vi "AlGaInPAs_prep_run_cont_dil_v16.vi"(2 "Debug Mode":bool, 3 "Elapsed Time(s)":dbl, 4 "State":enum16{"Edit", "Start", "Run", "End", "Idle"}(ring), 5 "Argument List In":string[](array[string])) -> (0 "Status Out":string, 1 "Argument List Out":string[](array[string]))   [LabVIEW 2011]
panel:
  out "Ga calculated var":u16(ring)=1 items=["Ga flow", "MFC1", "MFC2", "MFC3"]
  out "GAMFC3 var":dbl=100.0 caption="R3 (0-1000 sscm)" format="%.1f"
  out "GAMFC2 var":dbl=10.0 caption="R2 (0-100 sscm)" format="%.2f"
  out "GAMFC1 var":dbl=1.0 caption="R1 (0-10 sscm)" format="%.2f"
  out "Ga Flow var":dbl=1.0 caption="Ga Flow (0-10 sscm)" format="%.4f"
  out "Prep-In var":bool
  out "Prep-Ga var":bool
  out "Prep-Al var":bool
  out "Prep-P var":bool
  out "Prep-As var":bool
  out "prep_done":bool
  out "run started":bool
  out "first":bool=TRUE
  out "total time":dbl
  out "is OK?":bool
  out "AsH3?":bool
  out "PH3?":bool
  out "In?":bool
  out "Ga?":bool
  out "Al?":bool
  in  "Prep As":bool caption="Pre-run"
  in  "Prep P":bool caption="Pre-run"
  in  "Prep In":bool caption="Pre-run"
  in  "prep_time":dbl caption="pre-run time (s)"
  in  "Prep Al":bool caption="Pre-run"
  in  "Run As":bool caption="Run"
  in  "AsH3 Flow":dbl caption="AsH3 Flow (0-10 sccm)" format="%.2f"
  in  "P Flow":dbl caption="P Flow (0-100 sccm)" format="%.2f"
  in  "Run P":bool caption="Run"
  in  "In Flow":dbl caption="In Flow (0-100 sscm)" format="%.2f"
  in  "Run In":bool caption="Run"
  in  "Run Al":bool caption="Run"
  in  "Al Flow":dbl caption="Al Flow (0-100 sscm)" format="%.2f"
  in  "Cancel":bool
  in  "OK":bool
  out "tTotal(s) 2":dbl
  in  "Ga Tab Control":enum32{"Page 1", "Page 2", "Page 3"}(tab)
  in  "Ga Dilution":bool caption="Dilute"
  in  "Run Ga":bool caption="Run"
  in  "Prep Ga":bool caption="Pre-run"
  out "Ga Flow val":dbl=1.0 caption="Ga Flow (0-10 sscm)" format="%.4f"
  in  "Ga Flow set":dbl=1.0 caption="Ga Flow (0-10 sscm)" format="%.4f"
  out "GAMFC1 val":dbl=1.0 caption="R1 (0-10 sscm)" format="%.2f"
  out "GAMFC3 val":dbl=100.0 caption="R3 (0-1000 sscm)" format="%.1f"
  out "GAMFC2 val":dbl=10.0 caption="R2 (0-100 sscm)" format="%.2f"
  in  "GAMFC1 set":dbl=1.0 caption="R1 (0-10 sscm)" format="%.2f"
  in  "GAMFC2 set":dbl=10.0 caption="R2 (0-100 sscm)" format="%.2f"
  in  "GAMFC3 set":dbl=100.0 caption="R3 (0-1000 sscm)" format="%.1f"
  in  "Ga calculated":u16(ring)=1 items=["Ga flow", "MFC1", "MFC2", "MFC3"]
  # "Add pre-run time to run time in editor."
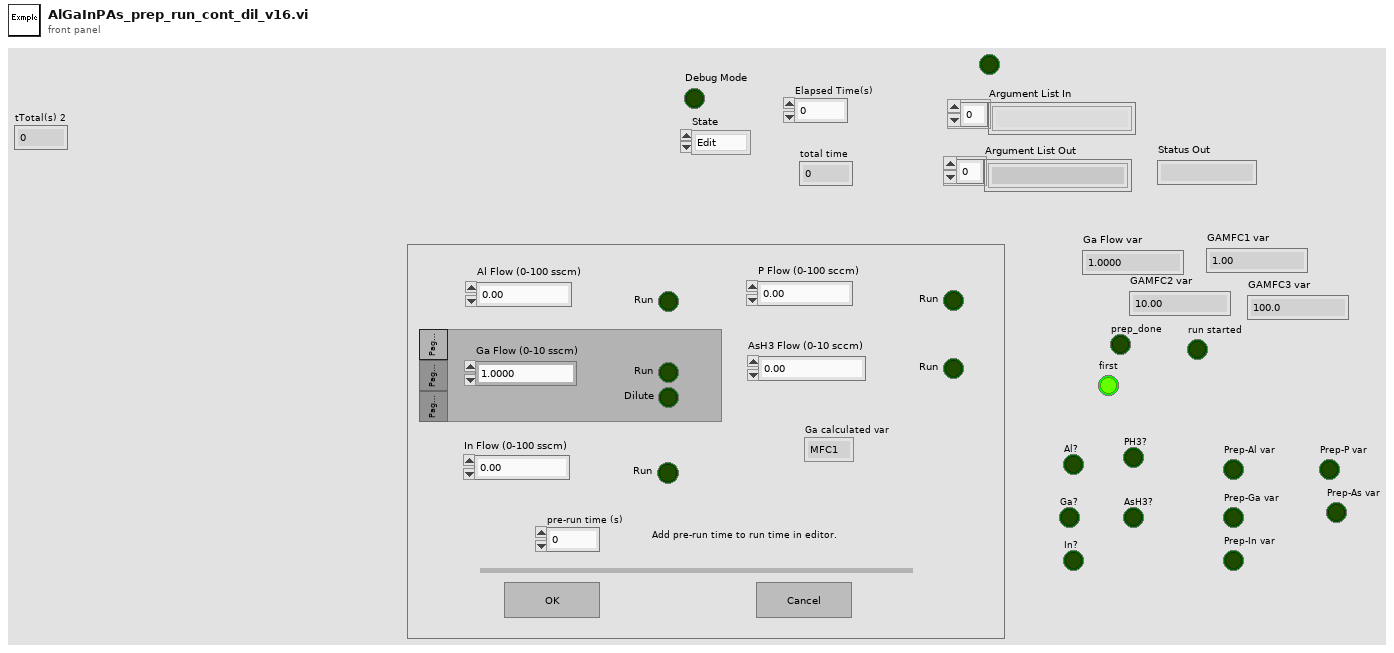
[diagram p1: front panel]
types:
  T1 = enum16{"Discrete", "Continuous", "Instantaneous", "Finite"}
  T2 = enum32{"Invalid", "Default", "Floating", "Floating/Auto-Hide", "Modal"}
  T3 = cluster{"Ga val":bool, "MFC1 val":bool, "MFC2 val":bool, "MFC3 val":bool, "Ga set":bool, "MFC1 set":bool, "MFC2 set":bool, "MFC3 set":bool}
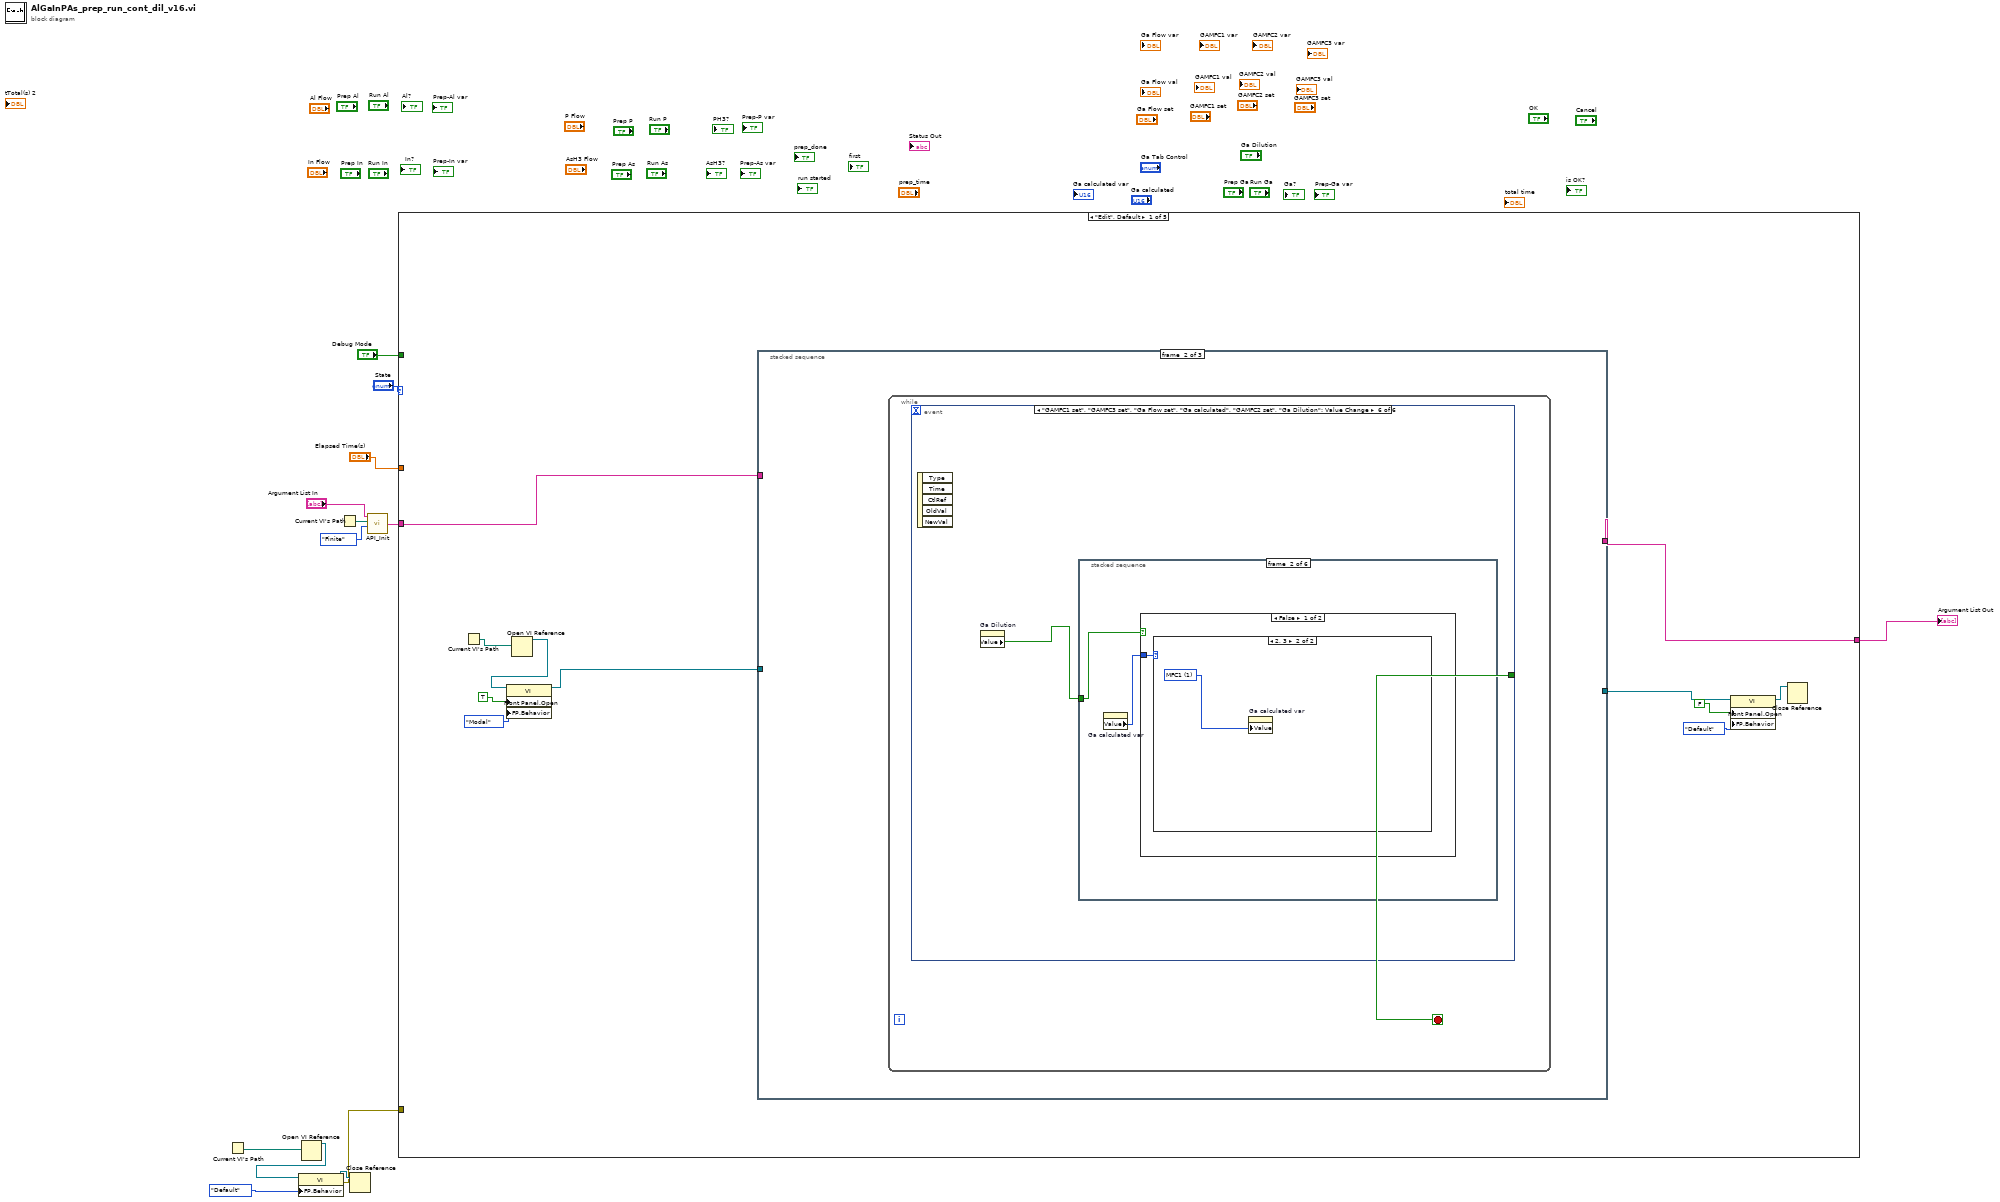
[diagram p0: block diagram]
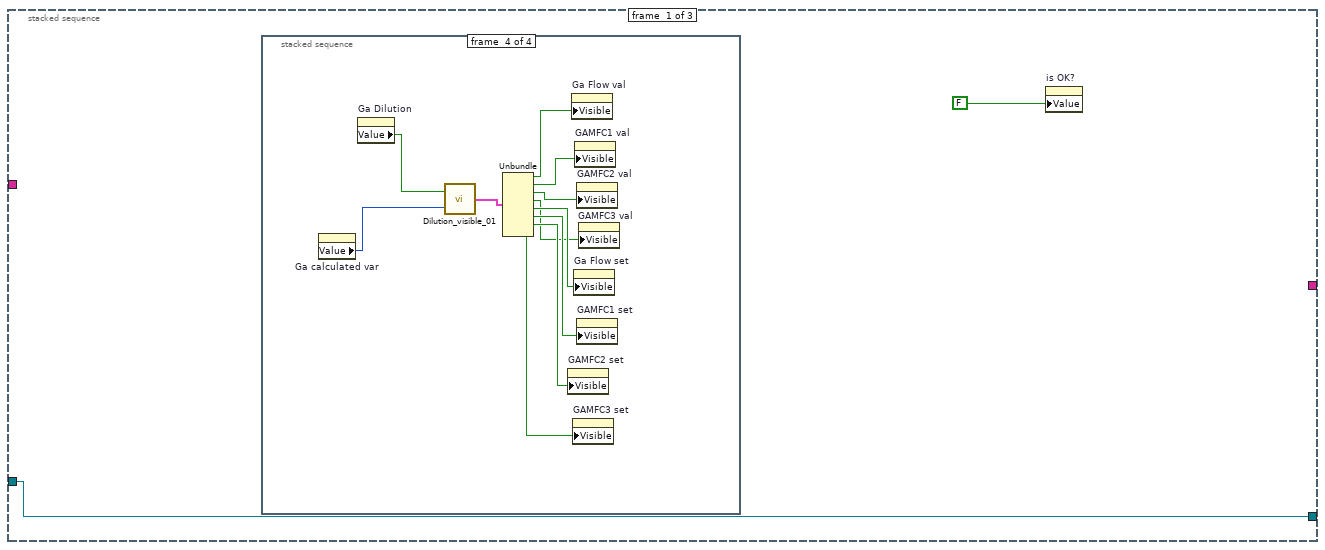
[diagram p2: hidden frame]
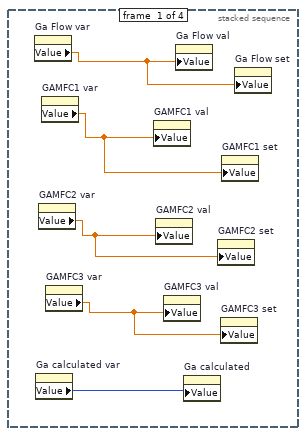
[diagram p3: hidden frame]
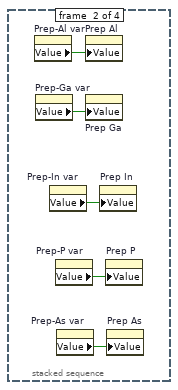
[diagram p4: hidden frame]
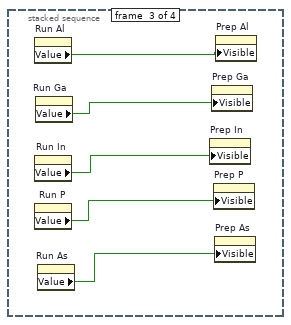
[diagram p5: hidden frame]
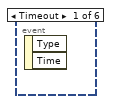
[diagram p6: hidden frame]
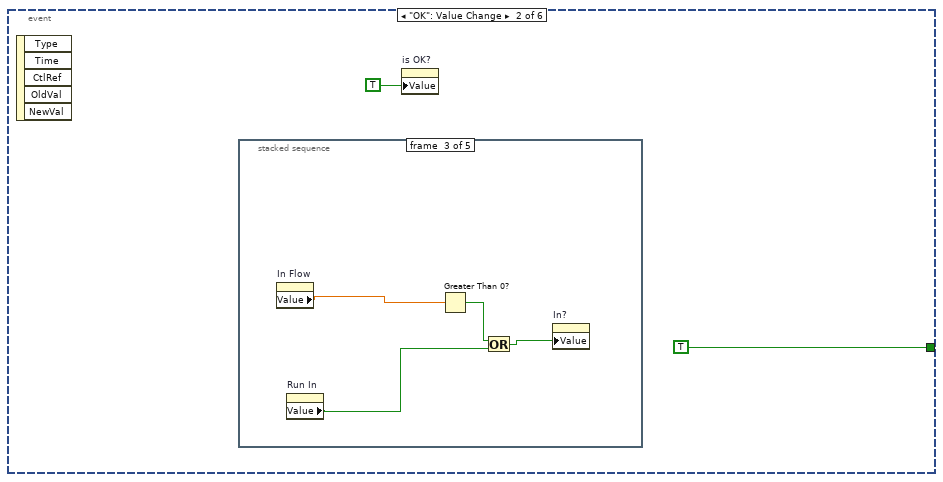
[diagram p7: hidden frame]
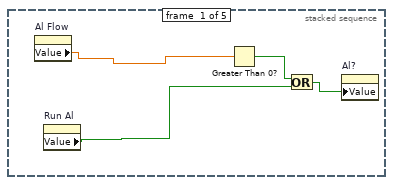
[diagram p8: hidden frame]
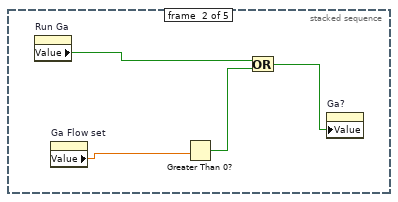
[diagram p9: hidden frame]
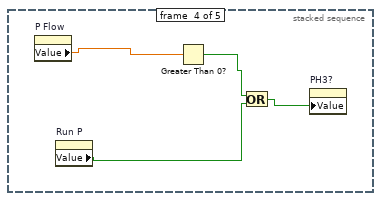
[diagram p10: hidden frame]
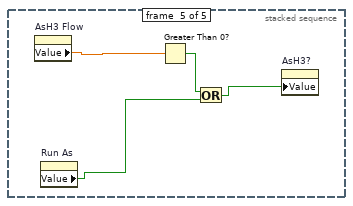
[diagram p11: hidden frame]
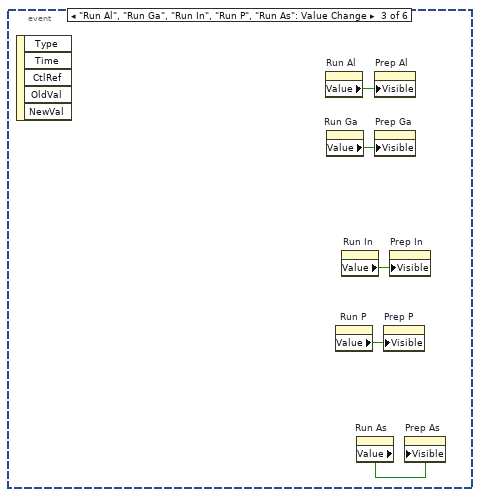
[diagram p12: hidden frame]
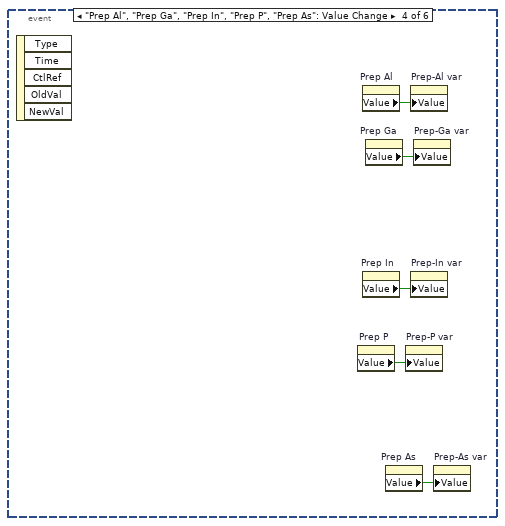
[diagram p13: hidden frame]
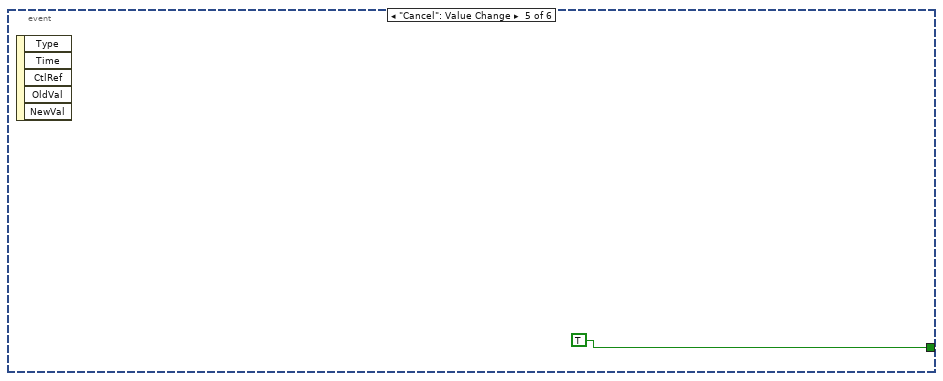
[diagram p14: hidden frame]
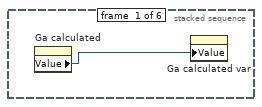
[diagram p15: hidden frame]
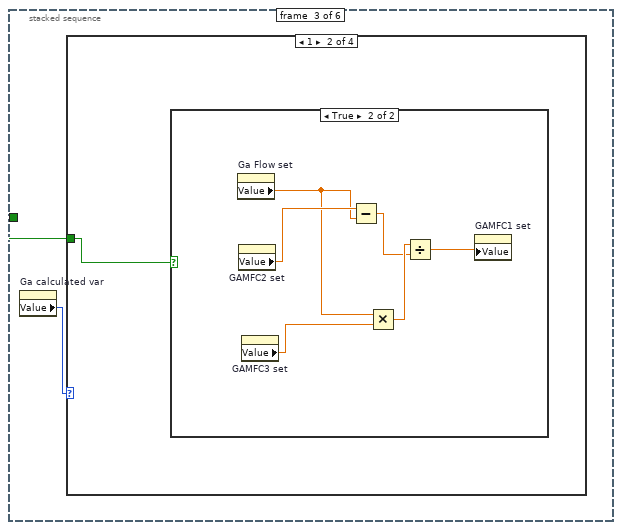
[diagram p18: hidden frame]
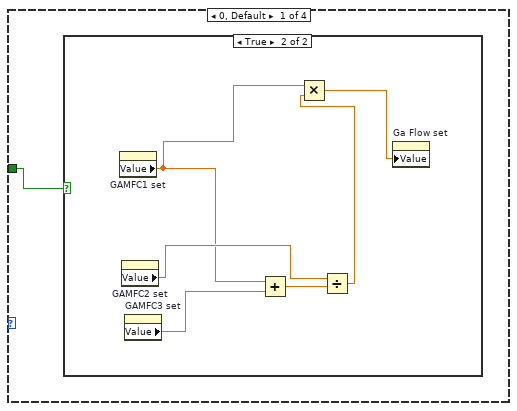
[diagram p19: hidden frame]
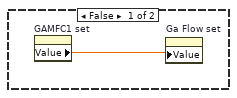
[diagram p20: hidden frame]
diagram:
  n1 = Current VI's Path() -> (path=w9:path)
  n2 = Open VI Reference(vi path=w9) -> (vi reference=w8:refnum<vi>)  [unwired: 1 in, 5 out]
  n3 = property class="VI"(reference=w8, "FP.Behavior"=T2."Default" ("Front Panel Window:Behavior")) -> (reference out=w6:refnum<vi>, error out=w5:errorcluster)  [unwired: 1 in]
  n4 = Current VI's Path() -> (path=w4:path)
  n5 = Close Reference(reference=w6) -> ()  [unwired: 1 in, 1 out]
  n6 = call "API_Init.vi"("API Mode"=T1."Finite", "VI Path"=w4, "Argument List In"="Argument List In") -> ("Argument List Out"=w1:string[])  [unwired: 1 in]
  n7 = case shown="\"Edit\", Default" "State" {
    tunnel: "Debug Mode" -> [_ w152 w206 _ _]
    tunnel: "Elapsed Time(s)" -> [_ _ w208 _ _]
    tunnel: w1 -> [w15 w154 w205 w323 w324]
    tunnel: [w14 w153 w207 w323 w324] -> w10
    tunnel: w5 -> [_ _ _ _ _]
    frame "Edit", Default {
      n8 = Current VI's Path() -> (path=w20:path)
      n9 = Open VI Reference(vi path=w20) -> (vi reference=w19:refnum<vi>)  [unwired: 1 in, 5 out]
      n10 = property class="VI"(reference=w19, "Front Panel.Open"=TRUE ("Front Panel Window:Open"), "FP.Behavior"=T2."Modal" ("Front Panel Window:Behavior")) -> (reference out=w18:refnum<vi>)  [unwired: 1 in, 1 out]
      n11 = stacked-sequence {
        tunnel: w15 -> [_ _ w147]
        tunnel: w18 -> [w26 _ _]
        tunnel: [w26 _ _] -> w22
        tunnel: [_ _ w145] -> w14
        frame #0 {
          n12 = stacked-sequence {
            frame #0 {
              n13 = property on="Ga Flow var" class="DigNum (strict)"() -> ("Value"=w31:dbl)  [unwired: 2 in, 2 out]
              n14 = property on="Ga calculated var" class="Ring (strict)"() -> ("Value"=w27:u16)  [unwired: 2 in, 2 out]
              n15 = property on="GAMFC2 var" class="DigNum (strict)"() -> ("Value"=w29:dbl)  [unwired: 2 in, 2 out]
              n16 = property on="GAMFC1 var" class="DigNum (strict)"() -> ("Value"=w28:dbl)  [unwired: 2 in, 2 out]
              n17 = property on="GAMFC3 var" class="DigNum (strict)"() -> ("Value"=w30:dbl)  [unwired: 2 in, 2 out]
              n18 = property on="GAMFC1 val" class="DigNum (strict)"("Value"=w28) -> ()  [unwired: 2 in, 2 out]
              n19 = property on="GAMFC2 val" class="DigNum (strict)"("Value"=w29) -> ()  [unwired: 2 in, 2 out]
              n20 = property on="GAMFC3 val" class="DigNum (strict)"("Value"=w30) -> ()  [unwired: 2 in, 2 out]
              n21 = property on="Ga Flow val" class="DigNum (strict)"("Value"=w31) -> ()  [unwired: 2 in, 2 out]
              n22 = property on="Ga calculated" class="Ring (strict)"("Value"=w27) -> ()  [unwired: 2 in, 2 out]
              n23 = property on="GAMFC2 set" class="DigNum (strict)"("Value"=w29) -> ()  [unwired: 2 in, 2 out]
              n24 = property on="GAMFC3 set" class="DigNum (strict)"("Value"=w30) -> ()  [unwired: 2 in, 2 out]
              n25 = property on="GAMFC1 set" class="DigNum (strict)"("Value"=w28) -> ()  [unwired: 2 in, 2 out]
              n26 = property on="Ga Flow set" class="DigNum (strict)"("Value"=w31) -> ()  [unwired: 2 in, 2 out]
            }
            frame #1 {
              n27 = property on="Prep-Al var" class="Bool (strict)"() -> ("Value"=w36:bool)  [unwired: 2 in, 2 out]
              n28 = property on="Prep-Ga var" class="Bool (strict)"() -> ("Value"=w35:bool)  [unwired: 2 in, 2 out]
              n29 = property on="Prep-In var" class="Bool (strict)"() -> ("Value"=w34:bool)  [unwired: 2 in, 2 out]
              n30 = property on="Prep-P var" class="Bool (strict)"() -> ("Value"=w33:bool)  [unwired: 2 in, 2 out]
              n31 = property on="Prep-As var" class="Bool (strict)"() -> ("Value"=w32:bool)  [unwired: 2 in, 2 out]
              n32 = property on="Prep Al" class="Bool (strict)"("Value"=w36) -> ()  [unwired: 2 in, 2 out]
              n33 = property on="Prep Ga" class="Bool (strict)"("Value"=w35) -> ()  [unwired: 2 in, 2 out]
              n34 = property on="Prep In" class="Bool (strict)"("Value"=w34) -> ()  [unwired: 2 in, 2 out]
              n35 = property on="Prep P" class="Bool (strict)"("Value"=w33) -> ()  [unwired: 2 in, 2 out]
              n36 = property on="Prep As" class="Bool (strict)"("Value"=w32) -> ()  [unwired: 2 in, 2 out]
            }
            frame #2 {
              n37 = property on="Run Al" class="Bool (strict)"() -> ("Value"=w41:bool)  [unwired: 2 in, 2 out]
              n38 = property on="Run In" class="Bool (strict)"() -> ("Value"=w39:bool)  [unwired: 2 in, 2 out]
              n39 = property on="Run P" class="Bool (strict)"() -> ("Value"=w38:bool)  [unwired: 2 in, 2 out]
              n40 = property on="Run Ga" class="Bool (strict)"() -> ("Value"=w40:bool)  [unwired: 2 in, 2 out]
              n41 = property on="Run As" class="Bool (strict)"() -> ("Value"=w37:bool)  [unwired: 2 in, 2 out]
              n42 = property on="Prep In" class="Bool (strict)"("Visible"=w39) -> ()  [unwired: 2 in, 2 out]
              n43 = property on="Prep Ga" class="Bool (strict)"("Visible"=w40) -> ()  [unwired: 2 in, 2 out]
              n44 = property on="Prep P" class="Bool (strict)"("Visible"=w38) -> ()  [unwired: 2 in, 2 out]
              n45 = property on="Prep As" class="Bool (strict)"("Visible"=w37) -> ()  [unwired: 2 in, 2 out]
              n46 = property on="Prep Al" class="Bool (strict)"("Visible"=w41) -> ()  [unwired: 2 in, 2 out]
            }
            frame #3 {
              n47 = property on="Ga calculated var" class="Ring (strict)"() -> ("Value"=w52:u16)  [unwired: 2 in, 2 out]
              n48 = property on="Ga Dilution" class="Bool (strict)"() -> ("Value"=w51:bool)  [unwired: 2 in, 2 out]
              n49 = call "Dilution_visible_01.vi"("calculated"=w52, "dilution"=w51) -> ("Visible"=w43:T3)
              n50 = Unbundle(w43) -> ("Ga val"=w44:bool, "MFC1 val"=w45:bool, "MFC2 val"=w42:bool, "MFC3 val"=w46:bool, "Ga set"=w47:bool, "MFC1 set"=w48:bool, "MFC2 set"=w49:bool, "MFC3 set"=w50:bool)
              n51 = property on="GAMFC2 set" class="DigNum (strict)"("Visible"=w49) -> ()  [unwired: 2 in, 2 out]
              n52 = property on="Ga Flow val" class="DigNum (strict)"("Visible"=w44) -> ()  [unwired: 2 in, 2 out]
              n53 = property on="GAMFC3 set" class="DigNum (strict)"("Visible"=w50) -> ()  [unwired: 2 in, 2 out]
              n54 = property on="Ga Flow set" class="DigNum (strict)"("Visible"=w47) -> ()  [unwired: 2 in, 2 out]
              n55 = property on="GAMFC1 val" class="DigNum (strict)"("Visible"=w45) -> ()  [unwired: 2 in, 2 out]
              n56 = property on="GAMFC2 val" class="DigNum (strict)"("Visible"=w42) -> ()  [unwired: 2 in, 2 out]
              n57 = property on="GAMFC1 set" class="DigNum (strict)"("Visible"=w48) -> ()  [unwired: 2 in, 2 out]
              n58 = property on="GAMFC3 val" class="DigNum (strict)"("Visible"=w46) -> ()  [unwired: 2 in, 2 out]
            }
          }
          n59 = property on="is OK?" class="Bool (strict)"("Value"=FALSE ("is OK?")) -> ()  [unwired: 2 in, 2 out]
        }
        frame #1 {
          n60 = while {
            stop <- w53 stop-if-true
            n61 = event shown="[5] \"GAMFC1 set\", \"GAMFC3 set\", \"Ga Flow set\", \"Ga calculated\", \"GAMFC2 set\", \"Ga Dilution\": Value Change" {
              selector: _ -> [_ _ _ _ _ _]
              dyn-events: _ -> [_ _ _ _ _ _]
              timeout: _ -> [_ _ _ _ _ _]
              tunnel: [_ TRUE _ _ TRUE _] -> w53
              event Timeout {
                n62 = event-data() -> ()  [unwired: 1 in, 2 out]
              }
              event "OK": Value Change {
                n63 = event-data() -> ()  [unwired: 1 in, 5 out]
                n64 = stacked-sequence {
                  frame #0 {
                    n65 = property on="Al Flow" class="DigNum (strict)"() -> ("Value"=w58:dbl)  [unwired: 2 in, 2 out]
                    n66 = property on="Run Al" class="Bool (strict)"() -> ("Value"=w57:bool)  [unwired: 2 in, 2 out]
                    n67 = Greater Than 0?(x=w58) -> (x > 0?=w59:bool)
                    n68 = Or(x=w59, y=w57) -> (x .or. y?=w56:bool)
                    n69 = property on="Al?" class="Bool (strict)"("Value"=w56) -> ()  [unwired: 2 in, 2 out]
                  }
                  frame #1 {
                    n70 = property on="Run Ga" class="Bool (strict)"() -> ("Value"=w61:bool)  [unwired: 2 in, 2 out]
                    n71 = property on="Ga Flow set" class="DigNum (strict)"() -> ("Value"=w62:dbl)  [unwired: 2 in, 2 out]
                    n72 = Greater Than 0?(x=w62) -> (x > 0?=w63:bool)
                    n73 = Or(x=w61, y=w63) -> (x .or. y?=w60:bool)
                    n74 = property on="Ga?" class="Bool (strict)"("Value"=w60) -> ()  [unwired: 2 in, 2 out]
                  }
                  frame #2 {
                    n75 = property on="In Flow" class="DigNum (strict)"() -> ("Value"=w65:dbl)  [unwired: 2 in, 2 out]
                    n76 = property on="Run In" class="Bool (strict)"() -> ("Value"=w66:bool)  [unwired: 2 in, 2 out]
                    n77 = Greater Than 0?(x=w65) -> (x > 0?=w67:bool)
                    n78 = Or(x=w67, y=w66) -> (x .or. y?=w64:bool)
                    n79 = property on="In?" class="Bool (strict)"("Value"=w64) -> ()  [unwired: 2 in, 2 out]
                  }
                  frame #3 {
                    n80 = property on="P Flow" class="DigNum (strict)"() -> ("Value"=w70:dbl)  [unwired: 2 in, 2 out]
                    n81 = property on="Run P" class="Bool (strict)"() -> ("Value"=w69:bool)  [unwired: 2 in, 2 out]
                    n82 = Greater Than 0?(x=w70) -> (x > 0?=w71:bool)
                    n83 = Or(x=w71, y=w69) -> (x .or. y?=w68:bool)
                    n84 = property on="PH3?" class="Bool (strict)"("Value"=w68) -> ()  [unwired: 2 in, 2 out]
                  }
                  frame #4 {
                    n85 = property on="AsH3 Flow" class="DigNum (strict)"() -> ("Value"=w74:dbl)  [unwired: 2 in, 2 out]
                    n86 = property on="Run As" class="Bool (strict)"() -> ("Value"=w73:bool)  [unwired: 2 in, 2 out]
                    n87 = Greater Than 0?(x=w74) -> (x > 0?=w75:bool)
                    n88 = Or(x=w75, y=w73) -> (x .or. y?=w72:bool)
                    n89 = property on="AsH3?" class="Bool (strict)"("Value"=w72) -> ()  [unwired: 2 in, 2 out]
                  }
                }
                n90 = property on="is OK?" class="Bool (strict)"("Value"=TRUE ("is OK?")) -> ()  [unwired: 2 in, 2 out]
              }
              event "Run Al", "Run Ga", "Run In", "Run P", "Run As": Value Change {
                n91 = event-data() -> ()  [unwired: 1 in, 5 out]
                n92 = property on="Run Al" class="Bool (strict)"() -> ("Value"=w80:bool)  [unwired: 2 in, 2 out]
                n93 = property on="Run Ga" class="Bool (strict)"() -> ("Value"=w79:bool)  [unwired: 2 in, 2 out]
                n94 = property on="Run P" class="Bool (strict)"() -> ("Value"=w76:bool)  [unwired: 2 in, 2 out]
                n95 = property on="Run In" class="Bool (strict)"() -> ("Value"=w78:bool)  [unwired: 2 in, 2 out]
                n96 = property on="Run As" class="Bool (strict)"() -> ("Value"=w77:bool)  [unwired: 2 in, 2 out]
                n97 = property on="Prep Al" class="Bool (strict)"("Visible"=w80) -> ()  [unwired: 2 in, 2 out]
                n98 = property on="Prep Ga" class="Bool (strict)"("Visible"=w79) -> ()  [unwired: 2 in, 2 out]
                n99 = property on="Prep P" class="Bool (strict)"("Visible"=w76) -> ()  [unwired: 2 in, 2 out]
                n100 = property on="Prep In" class="Bool (strict)"("Visible"=w78) -> ()  [unwired: 2 in, 2 out]
                n101 = property on="Prep As" class="Bool (strict)"("Visible"=w77) -> ()  [unwired: 2 in, 2 out]
              }
              event "Prep Al", "Prep Ga", "Prep In", "Prep P", "Prep As": Value Change {
                n102 = event-data() -> ()  [unwired: 1 in, 5 out]
                n103 = property on="Prep P" class="Bool (strict)"() -> ("Value"=w82:bool)  [unwired: 2 in, 2 out]
                n104 = property on="Prep Al" class="Bool (strict)"() -> ("Value"=w85:bool)  [unwired: 2 in, 2 out]
                n105 = property on="Prep In" class="Bool (strict)"() -> ("Value"=w83:bool)  [unwired: 2 in, 2 out]
                n106 = property on="Prep Ga" class="Bool (strict)"() -> ("Value"=w84:bool)  [unwired: 2 in, 2 out]
                n107 = property on="Prep As" class="Bool (strict)"() -> ("Value"=w81:bool)  [unwired: 2 in, 2 out]
                n108 = property on="Prep-P var" class="Bool (strict)"("Value"=w82) -> ()  [unwired: 2 in, 2 out]
                n109 = property on="Prep-Al var" class="Bool (strict)"("Value"=w85) -> ()  [unwired: 2 in, 2 out]
                n110 = property on="Prep-In var" class="Bool (strict)"("Value"=w83) -> ()  [unwired: 2 in, 2 out]
                n111 = property on="Prep-Ga var" class="Bool (strict)"("Value"=w84) -> ()  [unwired: 2 in, 2 out]
                n112 = property on="Prep-As var" class="Bool (strict)"("Value"=w81) -> ()  [unwired: 2 in, 2 out]
              }
              event "Cancel": Value Change {
                n113 = event-data() -> ()  [unwired: 1 in, 5 out]
              }
              event "GAMFC1 set", "GAMFC3 set", "Ga Flow set", "Ga calculated", "GAMFC2 set", "Ga Dilution": Value Change {
                n114 = event-data() -> ()  [unwired: 1 in, 5 out]
                n115 = property on="Ga Dilution" class="Bool (strict)"() -> ("Value"=w87:bool)  [unwired: 2 in, 2 out]
                n116 = stacked-sequence {
                  tunnel: w87 -> [_ w90 w94 w135 _ w141]
                  frame #0 {
                    n117 = property on="Ga calculated" class="Ring (strict)"() -> ("Value"=w88:u16)  [unwired: 2 in, 2 out]
                    n118 = property on="Ga calculated var" class="Ring (strict)"("Value"=w88) -> ()  [unwired: 2 in, 2 out]
                  }
                  frame #1 {
                    n119 = property on="Ga calculated var" class="Ring (strict)"() -> ("Value"=w89:u16)  [unwired: 2 in, 2 out]
                    n120 = case shown="False" w90 {
                      tunnel: w89 -> [w91 _]
                      frame False {
                        n121 = case shown="2, 3" w91 {
                          frame 0, 1, Default {
                          }
                          frame 2, 3 {
                            w92 = u16 1 items=["Ga flow", "MFC1", "MFC2", "MFC3"] ("Ga calculated")
                            n122 = property on="Ga calculated var" class="Ring (strict)"("Value"=w92) -> ()  [unwired: 2 in, 2 out]
                          }
                        }
                      }
                      frame True {
                      }
                    }
                  }
                  frame #2 {
                    n123 = property on="Ga calculated var" class="Ring (strict)"() -> ("Value"=w93:u16)  [unwired: 2 in, 2 out]
                    n124 = case shown="1" w93 {
                      tunnel: w94 -> [w95 w103 w111 w118]
                      frame 0, Default {
                        n125 = case shown="True" w95 {
                          frame False {
                            n126 = property on="GAMFC1 set" class="DigNum (strict)"() -> ("Value"=w96:dbl)  [unwired: 2 in, 2 out]
                            n127 = property on="Ga Flow set" class="DigNum (strict)"("Value"=w96) -> ()  [unwired: 2 in, 2 out]
                          }
                          frame True {
                            n128 = property on="GAMFC1 set" class="DigNum (strict)"() -> ("Value"=w98:dbl)  [unwired: 2 in, 2 out]
                            n129 = property on="GAMFC2 set" class="DigNum (strict)"() -> ("Value"=w100:dbl)  [unwired: 2 in, 2 out]
                            n130 = property on="GAMFC3 set" class="DigNum (strict)"() -> ("Value"=w102:dbl)  [unwired: 2 in, 2 out]
                            n131 = Add(x=w98, y=w102) -> (x+y=w101:dbl)
                            n132 = Divide(x=w100, y=w101) -> (x/y=w99:dbl)
                            n133 = Multiply(x=w98, y=w99) -> (x*y=w97:dbl)
                            n134 = property on="Ga Flow set" class="DigNum (strict)"("Value"=w97) -> ()  [unwired: 2 in, 2 out]
                          }
                        }
                      }
                      frame 1 {
                        n135 = case shown="True" w103 {
                          frame False {
                            n136 = property on="Ga Flow set" class="DigNum (strict)"() -> ("Value"=w104:dbl)  [unwired: 2 in, 2 out]
                            n137 = property on="GAMFC1 set" class="DigNum (strict)"("Value"=w104) -> ()  [unwired: 2 in, 2 out]
                          }
                          frame True {
                            n138 = property on="Ga Flow set" class="DigNum (strict)"() -> ("Value"=w109:dbl)  [unwired: 2 in, 2 out]
                            n139 = property on="GAMFC2 set" class="DigNum (strict)"() -> ("Value"=w110:dbl)  [unwired: 2 in, 2 out]
                            n140 = property on="GAMFC3 set" class="DigNum (strict)"() -> ("Value"=w108:dbl)  [unwired: 2 in, 2 out]
                            n141 = Subtract(x=w110, y=w109) -> (x-y=w106:dbl)
                            n142 = Multiply(x=w109, y=w108) -> (x*y=w107:dbl)
                            n143 = Divide(x=w107, y=w106) -> (x/y=w105:dbl)
                            n144 = property on="GAMFC1 set" class="DigNum (strict)"("Value"=w105) -> ()  [unwired: 2 in, 2 out]
                          }
                        }
                      }
                      frame 2 {
                        n145 = case shown="True" w111 {
                          frame False {
                          }
                          frame True {
                            n146 = property on="GAMFC1 set" class="DigNum (strict)"() -> ("Value"=w113:dbl)  [unwired: 2 in, 2 out]
                            n147 = property on="GAMFC3 set" class="DigNum (strict)"() -> ("Value"=w115:dbl)  [unwired: 2 in, 2 out]
                            n148 = property on="Ga Flow set" class="DigNum (strict)"() -> ("Value"=w116:dbl)  [unwired: 2 in, 2 out]
                            n149 = Add(x=w113, y=w115) -> (x+y=w117:dbl)
                            n150 = Multiply(x=w116, y=w117) -> (x*y=w114:dbl)
                            n151 = Divide(x=w114, y=w113) -> (x/y=w112:dbl)
                            n152 = property on="GAMFC2 set" class="DigNum (strict)"("Value"=w112) -> ()  [unwired: 2 in, 2 out]
                          }
                        }
                      }
                      frame 3 {
                        n153 = case shown="True" w118 {
                          frame False {
                          }
                          frame True {
                            n154 = property on="GAMFC2 set" class="DigNum (strict)"() -> ("Value"=w124:dbl)  [unwired: 2 in, 2 out]
                            n155 = property on="Ga Flow set" class="DigNum (strict)"() -> ("Value"=w122:dbl)  [unwired: 2 in, 2 out]
                            n156 = property on="GAMFC1 set" class="DigNum (strict)"() -> ("Value"=w123:dbl)  [unwired: 2 in, 2 out]
                            n157 = Subtract(x=w124, y=w122) -> (x-y=w120:dbl)
                            n158 = Divide(x=w123, y=w122) -> (x/y=w121:dbl)
                            n159 = Multiply(x=w121, y=w120) -> (x*y=w119:dbl)
                            n160 = property on="GAMFC3 set" class="DigNum (strict)"("Value"=w119) -> ()  [unwired: 2 in, 2 out]
                          }
                        }
                      }
                    }
                  }
                  frame #3 {
                    n161 = property on="Ga calculated var" class="Ring (strict)"() -> ("Value"=w125:u16)  [unwired: 2 in, 2 out]
                    n162 = call "Dilution_visible_01.vi"("calculated"=w125, "dilution"=w135) -> ("Visible"=w131:T3)
                    n163 = Unbundle(w131) -> ("Ga val"=w134:bool, "MFC1 val"=w133:bool, "MFC2 val"=w132:bool, "MFC3 val"=w130:bool, "Ga set"=w129:bool, "MFC1 set"=w128:bool, "MFC2 set"=w127:bool, "MFC3 set"=w126:bool)
                    n164 = property on="Ga Flow set" class="DigNum (strict)"("Visible"=w129) -> ()  [unwired: 2 in, 2 out]
                    n165 = property on="GAMFC1 set" class="DigNum (strict)"("Visible"=w128) -> ()  [unwired: 2 in, 2 out]
                    n166 = property on="GAMFC3 set" class="DigNum (strict)"("Visible"=w126) -> ()  [unwired: 2 in, 2 out]
                    n167 = property on="GAMFC2 set" class="DigNum (strict)"("Visible"=w127) -> ()  [unwired: 2 in, 2 out]
                    n168 = property on="Ga Flow val" class="DigNum (strict)"("Visible"=w134) -> ()  [unwired: 2 in, 2 out]
                    n169 = property on="GAMFC1 val" class="DigNum (strict)"("Visible"=w133) -> ()  [unwired: 2 in, 2 out]
                    n170 = property on="GAMFC2 val" class="DigNum (strict)"("Visible"=w132) -> ()  [unwired: 2 in, 2 out]
                    n171 = property on="GAMFC3 val" class="DigNum (strict)"("Visible"=w130) -> ()  [unwired: 2 in, 2 out]
                  }
                  frame #4 {
                    n172 = property on="GAMFC1 set" class="DigNum (strict)"() -> ("Value"=w139:dbl)  [unwired: 2 in, 2 out]
                    n173 = property on="Ga Flow set" class="DigNum (strict)"() -> ("Value"=w140:dbl)  [unwired: 2 in, 2 out]
                    n174 = property on="GAMFC2 set" class="DigNum (strict)"() -> ("Value"=w138:dbl)  [unwired: 2 in, 2 out]
                    n175 = property on="GAMFC3 set" class="DigNum (strict)"() -> ("Value"=w137:dbl)  [unwired: 2 in, 2 out]
                    n176 = property on="Ga calculated var" class="Ring (strict)"() -> ("Value"=w136:u16)  [unwired: 2 in, 2 out]
                    n177 = property on="GAMFC3 val" class="DigNum (strict)"("Value"=w137) -> ()  [unwired: 2 in, 2 out]
                    n178 = property on="GAMFC1 val" class="DigNum (strict)"("Value"=w139) -> ()  [unwired: 2 in, 2 out]
                    n179 = property on="GAMFC2 val" class="DigNum (strict)"("Value"=w138) -> ()  [unwired: 2 in, 2 out]
                    n180 = property on="Ga Flow val" class="DigNum (strict)"("Value"=w140) -> ()  [unwired: 2 in, 2 out]
                    n181 = property on="Ga calculated" class="Ring (strict)"("Value"=w136) -> ()  [unwired: 2 in, 2 out]
                    n182 = property on="GAMFC3 var" class="DigNum (strict)"("Value"=w137) -> ()  [unwired: 2 in, 2 out]
                    n183 = property on="GAMFC1 var" class="DigNum (strict)"("Value"=w139) -> ()  [unwired: 2 in, 2 out]
                    n184 = property on="GAMFC2 var" class="DigNum (strict)"("Value"=w138) -> ()  [unwired: 2 in, 2 out]
                    n185 = property on="Ga Flow var" class="DigNum (strict)"("Value"=w140) -> ()  [unwired: 2 in, 2 out]
                  }
                  frame #5 {
                    n186 = case shown="False" w141 {
                      frame False {
                        n187 = property on="Ga calculated" class="Ring (strict)"("Disabled Items []"=i32[] [2, 3]) -> ()  [unwired: 2 in, 2 out]
                      }
                      frame True {
                        n188 = property on="Ga calculated" class="Ring (strict)"("Disabled Items []"=i32[] []) -> ()  [unwired: 2 in, 2 out]
                      }
                    }
                  }
                }
              }
            }
          }
        }
        frame #2 {
          n189 = property on="is OK?" class="Bool (strict)"() -> ("Value"=w144:bool)  [unwired: 2 in, 2 out]
          n190 = case shown="True" w144 {
            tunnel: w147 -> [w150 w151]
            tunnel: [w150 w151] -> w146
            frame False {
            }
            frame True {
            }
          }
          n191 = Not(x=w144) -> (.not. x?=w149:bool)
          n192 = Current VI's Path() -> (path=w148:path)
          n193 = call "API_Edit.vi"("Cancel"=w149, "OK"=w144, "VI Path"=w148, "Argument List In"=w146) -> ("Argument List Out"=w145:string[])
        }
      }
      n194 = property class="VI"(reference=w22, "Front Panel.Open"=FALSE ("Front Panel Window:Open"), "FP.Behavior"=T2."Default" ("Front Panel Window:Behavior")) -> (reference out=w23:refnum<vi>)  [unwired: 1 in, 1 out]
      n195 = Close Reference(reference=w23) -> ()  [unwired: 1 in, 1 out]
    }
    frame "Start" {
      n196 = call "Set_Argument.vi"("Enable"=FALSE, "Argument"="run_started", "Argument List In"=w154) -> ("Argument List Out"=w153:string[])
      n197 = stacked-sequence {
        tunnel: w152 -> [w157 w166 w178 w187 w196]
        frame #0 {
          n198 = case shown="False" w157 {
            frame False {
              n199 = property on="Al?" class="Bool (strict)"() -> ("Value"=w158:bool)  [unwired: 2 in, 2 out]
              n200 = case shown="True" w158 {
                frame False {
                  w159 = FALSE ("Al Active")
                  n201 = call "set_Al.vi"("Aluminum Flow"=0.0, "Al Remote"=w159, "Al Run"=w159, "Al Bubbler"=w159, "Al Active"=w159) -> ()  [unwired: 5 out]
                }
                frame True {
                  w165 = TRUE ("Al Active")
                  n202 = property on="Prep Al" class="Bool (strict)"() -> ("Value"=w163:bool)  [unwired: 2 in, 2 out]
                  n203 = property on="Run Al" class="Bool (strict)"() -> ("Value"=w162:bool)  [unwired: 2 in, 2 out]
                  n204 = property on="Al Flow" class="DigNum (strict)"() -> ("Value"=w164:dbl)  [unwired: 2 in, 2 out]
                  n205 = And(x=w163, y=w162) -> (x .and. y?=w161:bool)
                  n206 = call "set_Al.vi"("Aluminum Flow"=w164, "Al Run"=w161, "Al Bubbler"=w165, "Al Active"=w165) -> ()  [unwired: 1 in, 5 out]
                }
              }
            }
            frame True {
            }
          }
        }
        frame #1 {
          n207 = case shown="False" w166 {
            frame False {
              n208 = property on="Ga?" class="Bool (strict)"() -> ("Value"=w167:bool)  [unwired: 2 in, 2 out]
              n209 = case shown="True" w167 {
                frame False {
                  w169 = FALSE ("Ga Active")
                  w168 = 0.0 ("Ga Flow 1")
                  n210 = call "set_Ga.vi"("Ga Active"=w169, "Ga Flow 3"=w168, "Ga Flow 2"=w168, "Ga Flow 1"=w168, "Ga Bubbler"=w169, "Ga H2 Dilute"=w169, "Ga Run"=w169, "Ga Remote"=w169) -> ()  [unwired: 8 out]
                }
                frame True {
                  w173 = TRUE ("Ga Active")
                  n211 = property on="GAMFC3 var" class="DigNum (strict)"() -> ("Value"=w170:dbl)  [unwired: 2 in, 2 out]
                  n212 = property on="GAMFC2 var" class="DigNum (strict)"() -> ("Value"=w171:dbl)  [unwired: 2 in, 2 out]
                  n213 = property on="GAMFC1 var" class="DigNum (strict)"() -> ("Value"=w172:dbl)  [unwired: 2 in, 2 out]
                  n214 = property on="Prep-Ga var" class="Bool (strict)"() -> ("Value"=w174:bool)  [unwired: 2 in, 2 out]
                  n215 = property on="Run Ga" class="Bool (strict)"() -> ("Value"=w175:bool)  [unwired: 2 in, 2 out]
                  n216 = And(x=w174, y=w175) -> (x .and. y?=w177:bool)
                  n217 = property on="Ga Dilution" class="Bool (strict)"() -> ("Value"=w176:bool)  [unwired: 2 in, 2 out]
                  n218 = call "set_Ga.vi"("Ga Active"=w173, "Ga Flow 3"=w170, "Ga Flow 2"=w171, "Ga Flow 1"=w172, "Ga Bubbler"=w173, "Ga H2 Dilute"=w176, "Ga Run"=w177, "Ga Remote"=w173) -> ()  [unwired: 8 in]
                }
              }
            }
            frame True {
            }
          }
        }
        frame #2 {
          n219 = case shown="False" w178 {
            frame False {
              n220 = property on="In?" class="Bool (strict)"() -> ("Value"=w179:bool)  [unwired: 2 in, 2 out]
              n221 = case shown="True" w179 {
                frame False {
                  w181 = FALSE ("In Remote")
                  n222 = call "set_In.vi"("Indium Flow"=0.0, "In Remote"=w181, "In Run"=w181, "In Bubbler"=w181, "In Active"=w181) -> ()  [unwired: 5 out]
                }
                frame True {
                  w186 = TRUE ("In Run")
                  n223 = property on="Run In" class="Bool (strict)"() -> ("Value"=w183:bool)  [unwired: 2 in, 2 out]
                  n224 = property on="Prep In" class="Bool (strict)"() -> ("Value"=w184:bool)  [unwired: 2 in, 2 out]
                  n225 = And(x=w184, y=w183) -> (x .and. y?=w182:bool)
                  n226 = property on="In Flow" class="DigNum (strict)"() -> ("Value"=w185:dbl)  [unwired: 2 in, 2 out]
                  n227 = call "set_In.vi"("Indium Flow"=w185, "In Run"=w182, "In Bubbler"=w186, "In Active"=w186) -> ()  [unwired: 1 in, 5 out]
                }
              }
            }
            frame True {
            }
          }
        }
        frame #3 {
          n228 = case shown="False" w187 {
            frame False {
              n229 = property on="PH3?" class="Bool (strict)"() -> ("Value"=w188:bool)  [unwired: 2 in, 2 out]
              n230 = case shown="True" w188 {
                frame False {
                  w189 = FALSE ("P_Gas Active")
                  n231 = call "set_P_gas.vi"("P_Gas Active"=w189, "P_Gas Flow"=0.0, "P_Gas In"=w189, "P_Gas H2 In"=w189, "P_Gas Run"=w189, "P_Gas Remote"=w189) -> ()  [unwired: 10 out]
                }
                frame True {
                  w195 = TRUE ("P_Gas Active")
                  n232 = property on="P Flow" class="DigNum (strict)"() -> ("Value"=w194:dbl)  [unwired: 2 in, 2 out]
                  n233 = property on="Prep P" class="Bool (strict)"() -> ("Value"=w193:bool)  [unwired: 2 in, 2 out]
                  n234 = property on="Run P" class="Bool (strict)"() -> ("Value"=w192:bool)  [unwired: 2 in, 2 out]
                  n235 = And(x=w193, y=w192) -> (x .and. y?=w191:bool)
                  n236 = call "set_P_gas.vi"("P_Gas Active"=w195, "P_Gas Flow"=w194, "P_Gas In"=w195, "P_Gas Run"=w191) -> ()  [unwired: 2 in, 10 out]
                }
              }
            }
            frame True {
            }
          }
        }
        frame #4 {
          n237 = case shown="False" w196 {
            frame False {
              n238 = property on="AsH3?" class="Bool (strict)"() -> ("Value"=w197:bool)  [unwired: 2 in, 2 out]
              n239 = case shown="True" w197 {
                frame False {
                  w198 = FALSE ("As_Gas Active")
                  n240 = call "set_As_gas.vi"("As_Gas Active"=w198, "As_Gas Flow"=0.0, "As_Gas In"=w198, "As_Gas H2"=w198, "As_Gas Run"=w198, "As_Gas Remote"=w198) -> ()  [unwired: 10 in]
                }
                frame True {
                  w204 = TRUE ("As_Gas Active")
                  n241 = property on="Prep As" class="Bool (strict)"() -> ("Value"=w201:bool)  [unwired: 2 in, 2 out]
                  n242 = property on="Run As" class="Bool (strict)"() -> ("Value"=w202:bool)  [unwired: 2 in, 2 out]
                  n243 = property on="AsH3 Flow" class="DigNum (strict)"() -> ("Value"=w203:dbl)  [unwired: 2 in, 2 out]
                  n244 = And(x=w201, y=w202) -> (x .and. y?=w200:bool)
                  n245 = call "set_As_gas.vi"("As_Gas Active"=w204, "As_Gas Flow"=w203, "As_Gas In"=w204, "As_Gas Run"=w200) -> ()  [unwired: 12 in]
                }
              }
            }
            frame True {
            }
          }
        }
      }
    }
    frame "Run" {
      n246 = stacked-sequence {
        tunnel: w208 -> [_ w213 _ _]
        tunnel: w205 -> [w210 _ _ w267]
        tunnel: [_ _ _ w266] -> w207
        tunnel: w206 -> [_ _ _ w268]
        frame #0 {
          n247 = call "Get_Argument.vi"("Argument"="run_started", "Argument List"=w210) -> ("Enabled"=w209:bool)
          n248 = local write "run started"(w209) -> ()
        }
        frame #1 {
          n249 = property on="prep_time" class="DigNum (strict)"() -> ("Value"=w214:dbl)  [unwired: 2 in, 2 out]
          n250 = Greater Or Equal?(x=w213, y=w214) -> (x >= y?=w212:bool)
          n251 = local write "prep_done"(w212) -> ()
        }
        frame #2 {
          n252 = local read "run started"() -> (w216:bool)
          n253 = Not(x=w216) -> (.not. x?=w215:bool)
          n254 = stacked-sequence {
            tunnel: w215 -> [w218 w222 w231 w240 w249 w258]
            frame #0 {
              n255 = case shown="True" w218 {
                tunnel: ["run: " "pre-run: "] -> w217
                frame False {
                }
                frame True {
                }
              }
              n256 = property on="Status Out" class="Str"("Value"=w217) -> ()  [unwired: 2 in, 2 out]
            }
            frame #1 {
              n257 = property on="Status Out" class="Str"() -> ("Value"=w228:string)  [unwired: 2 in, 2 out]
              n258 = property on="Al?" class="Bool (strict)"() -> ("Value"=w229:bool)  [unwired: 2 in, 2 out]
              n259 = property on="Run Al" class="Bool (strict)"() -> ("Value"=w221:bool)  [unwired: 2 in, 2 out]
              n260 = property on="Prep Al" class="Bool (strict)"() -> ("Value"=w223:bool)  [unwired: 2 in, 2 out]
              n261 = call "flow_strings.vi"("string in"=w228, "is first in?"=TRUE, "use source?"=w229, "name"="Al", "run source?"=w221, "prep source?"=w223, "is prep?"=w222) -> ("string out"=w227:string, "is first out?"=w226:bool)
              n262 = property on="Status Out" class="Str"("Value"=w227) -> ()  [unwired: 2 in, 2 out]
              n263 = property on="first" class="Bool (strict)"("Value"=w226) -> ()  [unwired: 2 in, 2 out]
            }
            frame #2 {
              n264 = property on="first" class="Bool (strict)"() -> ("Value"=w234:bool)  [unwired: 2 in, 2 out]
              n265 = property on="Status Out" class="Str"() -> ("Value"=w237:string)  [unwired: 2 in, 2 out]
              n266 = property on="Ga?" class="Bool (strict)"() -> ("Value"=w235:bool)  [unwired: 2 in, 2 out]
              n267 = property on="Run Ga" class="Bool (strict)"() -> ("Value"=w230:bool)  [unwired: 2 in, 2 out]
              n268 = property on="Prep Ga" class="Bool (strict)"() -> ("Value"=w232:bool)  [unwired: 2 in, 2 out]
              n269 = call "flow_strings.vi"("string in"=w237, "is first in?"=w234, "use source?"=w235, "name"="Ga", "run source?"=w230, "prep source?"=w232, "is prep?"=w231) -> ("string out"=w238:string, "is first out?"=w233:bool)
              n270 = property on="Status Out" class="Str"("Value"=w238) -> ()  [unwired: 2 in, 2 out]
              n271 = property on="first" class="Bool (strict)"("Value"=w233) -> ()  [unwired: 2 in, 2 out]
            }
            frame #3 {
              n272 = property on="first" class="Bool (strict)"() -> ("Value"=w244:bool)  [unwired: 2 in, 2 out]
              n273 = property on="Status Out" class="Str"() -> ("Value"=w246:string)  [unwired: 2 in, 2 out]
              n274 = property on="In?" class="Bool (strict)"() -> ("Value"=w247:bool)  [unwired: 2 in, 2 out]
              n275 = property on="Run In" class="Bool (strict)"() -> ("Value"=w239:bool)  [unwired: 2 in, 2 out]
              n276 = property on="Prep In" class="Bool (strict)"() -> ("Value"=w241:bool)  [unwired: 2 in, 2 out]
              n277 = call "flow_strings.vi"("string in"=w246, "is first in?"=w244, "use source?"=w247, "name"="In", "run source?"=w239, "prep source?"=w241, "is prep?"=w240) -> ("string out"=w243:string, "is first out?"=w242:bool)
              n278 = property on="Status Out" class="Str"("Value"=w243) -> ()  [unwired: 2 in, 2 out]
              n279 = property on="first" class="Bool (strict)"("Value"=w242) -> ()  [unwired: 2 in, 2 out]
            }
            frame #4 {
              n280 = property on="first" class="Bool (strict)"() -> ("Value"=w252:bool)  [unwired: 2 in, 2 out]
              n281 = property on="Status Out" class="Str"() -> ("Value"=w254:string)  [unwired: 2 in, 2 out]
              n282 = property on="PH3?" class="Bool (strict)"() -> ("Value"=w255:bool)  [unwired: 2 in, 2 out]
              n283 = property on="Run P" class="Bool (strict)"() -> ("Value"=w248:bool)  [unwired: 2 in, 2 out]
              n284 = property on="Prep P" class="Bool (strict)"() -> ("Value"=w250:bool)  [unwired: 2 in, 2 out]
              n285 = call "flow_strings.vi"("string in"=w254, "is first in?"=w252, "use source?"=w255, "name"="P", "run source?"=w248, "prep source?"=w250, "is prep?"=w249) -> ("string out"=w253:string, "is first out?"=w251:bool)
              n286 = property on="Status Out" class="Str"("Value"=w253) -> ()  [unwired: 2 in, 2 out]
              n287 = property on="first" class="Bool (strict)"("Value"=w251) -> ()  [unwired: 2 in, 2 out]
            }
            frame #5 {
              n288 = property on="first" class="Bool (strict)"() -> ("Value"=w261:bool)  [unwired: 2 in, 2 out]
              n289 = property on="Status Out" class="Str"() -> ("Value"=w263:string)  [unwired: 2 in, 2 out]
              n290 = property on="AsH3?" class="Bool (strict)"() -> ("Value"=w264:bool)  [unwired: 2 in, 2 out]
              n291 = property on="Run As" class="Bool (strict)"() -> ("Value"=w257:bool)  [unwired: 2 in, 2 out]
              n292 = property on="Prep As" class="Bool (strict)"() -> ("Value"=w259:bool)  [unwired: 2 in, 2 out]
              n293 = call "flow_strings.vi"("string in"=w263, "is first in?"=w261, "use source?"=w264, "name"="As", "run source?"=w257, "prep source?"=w259, "is prep?"=w258) -> ("string out"=w260:string, "is first out?"=w262:bool)
              n294 = property on="Status Out" class="Str"("Value"=w260) -> ()  [unwired: 2 in, 2 out]
              n295 = property on="first" class="Bool (strict)"("Value"=w262) -> ()  [unwired: 2 in, 2 out]
            }
          }
        }
        frame #3 {
          n296 = local read "run started"() -> (w271:bool)
          n297 = local read "prep_done"() -> (w269:bool)
          n298 = Not(x=w271) -> (.not. x?=w272:bool)
          n299 = And(x=w269, y=w272) -> (x .and. y?=w270:bool)
          n300 = stacked-sequence {
            tunnel: w270 -> [w276]
            tunnel: w268 -> [w275]
            tunnel: w267 -> [w274]
            tunnel: [w273] -> w266
            frame #0 {
              n301 = case shown="True" w276 {
                tunnel: w275 -> [_ w280]
                tunnel: w274 -> [w277 w279]
                tunnel: [w277 w278] -> w273
                frame False {
                }
                frame True {
                  n302 = stacked-sequence {
                    tunnel: w280 -> [w281 w288 w298 w305 w312 _]
                    tunnel: w279 -> [_ _ _ _ _ w320]
                    tunnel: [_ _ _ _ _ w319] -> w278
                    frame #0 {
                      n303 = case shown="False" w281 {
                        frame False {
                          n304 = property on="Al?" class="Bool (strict)"() -> ("Value"=w282:bool)  [unwired: 2 in, 2 out]
                          n305 = case shown="True" w282 {
                            frame False {
                              w283 = FALSE ("Al Active")
                              n306 = call "set_Al.vi"("Aluminum Flow"=0.0, "Al Remote"=w283, "Al Run"=w283, "Al Bubbler"=w283, "Al Active"=w283) -> ()  [unwired: 5 out]
                            }
                            frame True {
                              w287 = TRUE ("Al Active")
                              n307 = property on="Al Flow" class="DigNum (strict)"() -> ("Value"=w286:dbl)  [unwired: 2 in, 2 out]
                              n308 = property on="Run Al" class="Bool (strict)"() -> ("Value"=w285:bool)  [unwired: 2 in, 2 out]
                              n309 = call "set_Al.vi"("Aluminum Flow"=w286, "Al Run"=w285, "Al Bubbler"=w287, "Al Active"=w287) -> ()  [unwired: 1 in, 5 out]
                            }
                          }
                        }
                        frame True {
                        }
                      }
                    }
                    frame #1 {
                      n310 = case shown="False" w288 {
                        frame False {
                          n311 = property on="Ga?" class="Bool (strict)"() -> ("Value"=w289:bool)  [unwired: 2 in, 2 out]
                          n312 = case shown="True" w289 {
                            frame False {
                              w291 = FALSE ("Ga Active")
                              w290 = 0.0 ("Ga Flow 1")
                              n313 = call "set_Ga.vi"("Ga Active"=w291, "Ga Flow 3"=w290, "Ga Flow 2"=w290, "Ga Flow 1"=w290, "Ga Bubbler"=w291, "Ga H2 Dilute"=w291, "Ga Run"=w291, "Ga Remote"=w291) -> ()  [unwired: 8 out]
                            }
                            frame True {
                              w295 = TRUE ("Ga Active")
                              n314 = property on="Ga Dilution" class="Bool (strict)"() -> ("Value"=w294:bool)  [unwired: 2 in, 2 out]
                              n315 = property on="GAMFC3 val" class="DigNum (strict)"() -> ("Value"=w293:dbl)  [unwired: 2 in, 2 out]
                              n316 = property on="Run Ga" class="Bool (strict)"() -> ("Value"=w296:bool)  [unwired: 2 in, 2 out]
                              n317 = property on="GAMFC2 val" class="DigNum (strict)"() -> ("Value"=w297:dbl)  [unwired: 2 in, 2 out]
                              n318 = property on="GAMFC1 val" class="DigNum (strict)"() -> ("Value"=w292:dbl)  [unwired: 2 in, 2 out]
                              n319 = call "set_Ga.vi"("Ga Active"=w295, "Ga Flow 3"=w293, "Ga Flow 2"=w297, "Ga Flow 1"=w292, "Ga Bubbler"=w295, "Ga H2 Dilute"=w294, "Ga Run"=w296, "Ga Remote"=w295) -> ()  [unwired: 8 in]
                            }
                          }
                        }
                        frame True {
                        }
                      }
                    }
                    frame #2 {
                      n320 = case shown="False" w298 {
                        frame False {
                          n321 = property on="In?" class="Bool (strict)"() -> ("Value"=w299:bool)  [unwired: 2 in, 2 out]
                          n322 = case shown="True" w299 {
                            frame False {
                              w301 = FALSE ("In Remote")
                              n323 = call "set_In.vi"("Indium Flow"=0.0, "In Remote"=w301, "In Run"=w301, "In Bubbler"=w301, "In Active"=w301) -> ()  [unwired: 5 out]
                            }
                            frame True {
                              w304 = TRUE ("In Run")
                              n324 = property on="Run In" class="Bool (strict)"() -> ("Value"=w302:bool)  [unwired: 2 in, 2 out]
                              n325 = property on="In Flow" class="DigNum (strict)"() -> ("Value"=w303:dbl)  [unwired: 2 in, 2 out]
                              n326 = call "set_In.vi"("Indium Flow"=w303, "In Run"=w302, "In Bubbler"=w304, "In Active"=w304) -> ()  [unwired: 1 in, 5 out]
                            }
                          }
                        }
                        frame True {
                        }
                      }
                    }
                    frame #3 {
                      n327 = case shown="False" w305 {
                        frame False {
                          n328 = property on="PH3?" class="Bool (strict)"() -> ("Value"=w306:bool)  [unwired: 2 in, 2 out]
                          n329 = case shown="False" w306 {
                            frame False {
                              w307 = FALSE ("P_Gas Active")
                              n330 = call "set_P_gas.vi"("P_Gas Active"=w307, "P_Gas Flow"=0.0, "P_Gas In"=w307, "P_Gas H2 In"=w307, "P_Gas Run"=w307, "P_Gas Remote"=w307) -> ()  [unwired: 10 out]
                            }
                            frame True {
                              w311 = TRUE ("P_Gas Active")
                              n331 = property on="P Flow" class="DigNum (strict)"() -> ("Value"=w310:dbl)  [unwired: 2 in, 2 out]
                              n332 = property on="Run P" class="Bool (strict)"() -> ("Value"=w309:bool)  [unwired: 2 in, 2 out]
                              n333 = call "set_P_gas.vi"("P_Gas Active"=w311, "P_Gas Flow"=w310, "P_Gas In"=w311, "P_Gas Run"=w309) -> ()  [unwired: 2 in, 10 out]
                            }
                          }
                        }
                        frame True {
                        }
                      }
                    }
                    frame #4 {
                      n334 = case shown="False" w312 {
                        frame False {
                          n335 = property on="AsH3?" class="Bool (strict)"() -> ("Value"=w313:bool)  [unwired: 2 in, 2 out]
                          n336 = case shown="True" w313 {
                            frame False {
                              w314 = FALSE ("As_Gas Active")
                              n337 = call "set_As_gas.vi"("As_Gas Active"=w314, "As_Gas Flow"=0.0, "As_Gas In"=w314, "As_Gas H2"=w314, "As_Gas Run"=w314, "As_Gas Remote"=w314) -> ()  [unwired: 10 in]
                            }
                            frame True {
                              w317 = TRUE ("As_Gas Active")
                              n338 = property on="Run As" class="Bool (strict)"() -> ("Value"=w316:bool)  [unwired: 2 in, 2 out]
                              n339 = property on="AsH3 Flow" class="DigNum (strict)"() -> ("Value"=w318:dbl)  [unwired: 2 in, 2 out]
                              n340 = call "set_As_gas.vi"("As_Gas Active"=w317, "As_Gas Flow"=w318, "As_Gas In"=w317, "As_Gas Run"=w316) -> ()  [unwired: 12 in]
                            }
                          }
                        }
                        frame True {
                        }
                      }
                    }
                    frame #5 {
                      n341 = call "Set_Argument.vi"("Enable"=TRUE, "Argument"="run_started", "Argument List In"=w320) -> ("Argument List Out"=w319:string[])
                    }
                  }
                }
              }
            }
          }
        }
      }
    }
    frame "End" {
    }
    frame "Idle" {
    }
  }
  "Argument List Out" <- w10
